vi "OutputRF.vi"(6 "Cal Routes":string[](array[string]), 7 "output enabled":bool=TRUE, 8 "error in (no error)":errorcluster, 9 "Power (dBm)":dbl, 10 "Frequency (Hz)":dbl, 11 "Instrument in":refnum<class "Instrument.lvclass">) -> (0 "error out":errorcluster, 3 "Instrument out":refnum<class "Instrument.lvclass">)   [LabVIEW 2014, in "Instrument.lvclass"]
uses:
  Instrument.lvclass
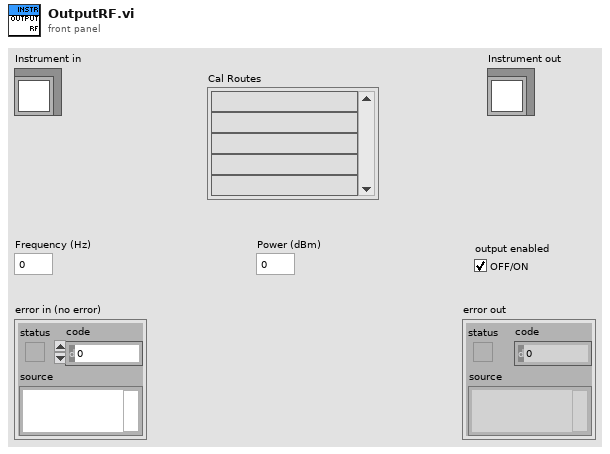
[diagram p1: front panel]
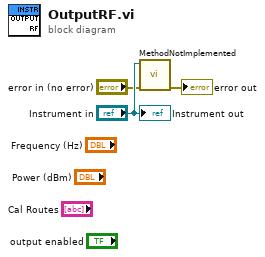
[diagram p0: block diagram]
diagram:
  n1 = call "MethodNotImplemented.vi"("error in (no error)"="error in (no error)", "LabVIEW Object In"="Instrument in") -> ("error out"=→"error out":errorcluster)  [unwired: 9 in]
  "Instrument out" <- "Instrument in"
